vi "Calculate Hypotenuse.vi"(1 "Y":dbl, 2 "X":dbl) -> (0 "Hypotenuse":dbl)   [LabVIEW 2016]
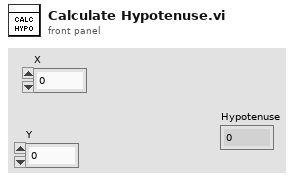
[diagram p1: front panel]
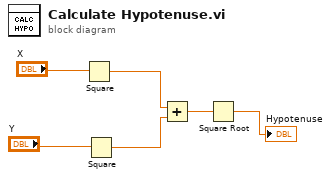
[diagram p0: block diagram]
diagram:
  n1 = Square(x="X") -> (x^2=w4:dbl)
  n2 = Square(x="Y") -> (x^2=w3:dbl)
  n3 = Add(x=w4, y=w3) -> (x+y=w2:dbl)
  n4 = Square Root(x=w2) -> (sqrt(x)=→"Hypotenuse":dbl)
